vi "GenILCTestProf.vi"() -> ()   [LabVIEW 2016]
panel:
  in  "Offset [deg or mm]":dbl
  out "RUY Signals":T1
  in  "No Cycles":u16=3
  in  "Dwell Time [s]":dbl=1.0
  in  "Max Speed [/s]":dbl=5.0
  in  "Travel [deg or mm]":dbl=20.0
  in  "Select Joint No.":T2(ring)=enum."Joint 3"
  out "Joint 4 Graph":dbl[](graph)
  out "Joint 3 Graph":dbl[](graph)
  out "Joint 2 Graph":dbl[](graph)
  out "Joint 1 Graph":dbl[](graph)
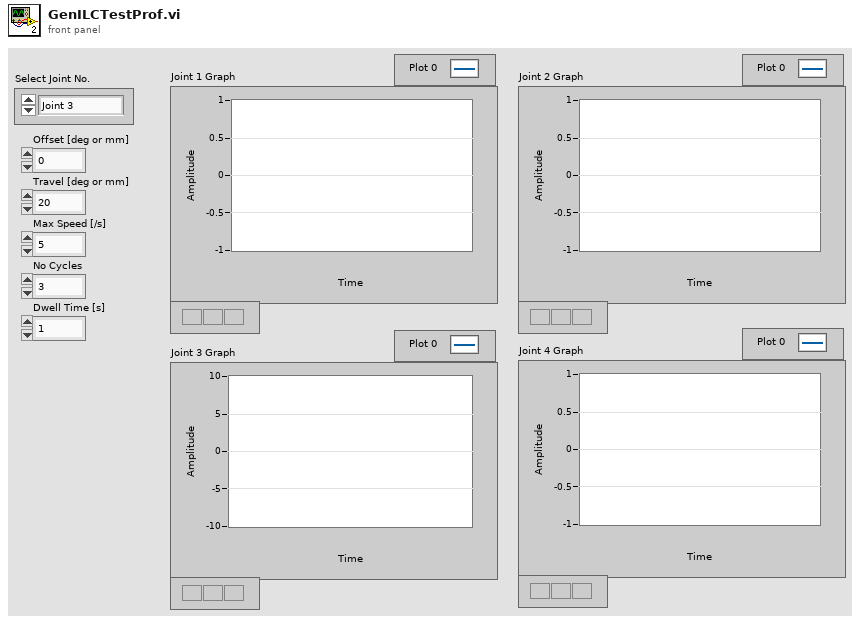
[diagram p1: front panel]
types:
  T1 = cluster{"Ref":cluster{"theta 1 Array":dbl[], "theta 2 Array":dbl[], "d3 Array":dbl[], "theta 4 Array":dbl[]}, "uFF":cluster{"theta 1 Array":dbl[], "theta 2 Array":dbl[], "d3 Array":dbl[], "theta 4 Array":dbl[]}, "yOut":cluster{"theta 1 Array":dbl[], "theta 2 Array":dbl[], "d3 Array":dbl[], "theta 4 Array":dbl[]}}
  T2 = enum16{"Joint 1", "Joint 2", "Joint 3", "Joint 4"}
  T3 = cluster{"theta 1 Array":dbl[], "theta 2 Array":dbl[], "d3 Array":dbl[], "theta 4 Array":dbl[]}
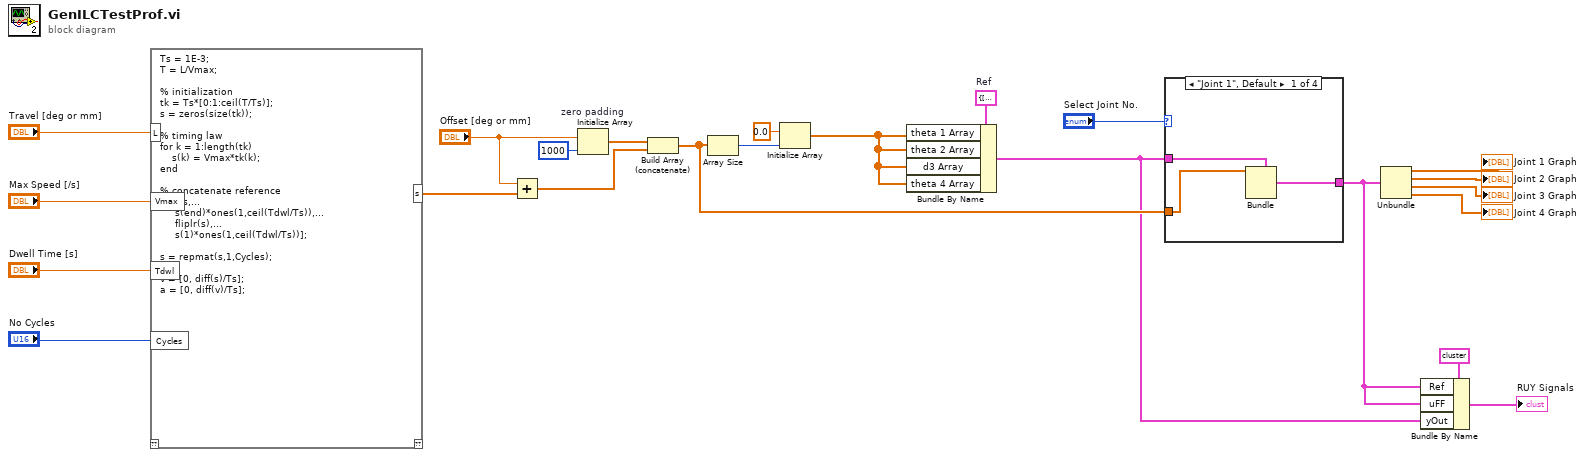
[diagram p0: block diagram]
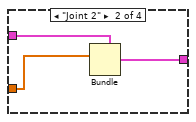
[diagram p2: hidden frame]
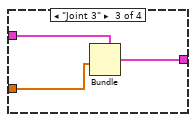
[diagram p3: hidden frame]
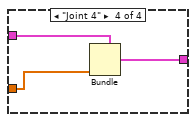
[diagram p4: hidden frame]
diagram:
  w15 = T3 {"theta 1 Array"=[], "theta 2 Array"=[], "d3 Array"=[], "theta 4 Array"=[]}  # Ref
  n1 = script code="Ts = 1E-3;\nT = L/Vmax;\n\n% initialization\ntk = Ts*[0:1:ceil(T/Ts)];\ns = zeros(size(tk));\n\n% timing law\nfor k = 1:length(tk) \n    s(k) = Vmax*tk(k);\nend\n\n% concatenate reference\ns = [s,...\n     s(end)*ones(1,ceil(Tdwl/Ts)),...\n     fliplr(s),...\n     s(1)*ones(1,ceil(Tdwl/Ts))];\n\ns = repmat(s,1,Cycles);\n\nv = [0, diff(s)/Ts];\na = [0, diff(v)/Ts];"("L"="Travel [deg or mm]", "Vmax"="Max Speed [/s]", "Tdwl"="Dwell Time [s]", "Cycles"="No Cycles") -> ("s"=w2:dbl[])  [unwired: 1 in, 1 out]
  n2 = Add(x="Offset [deg or mm]", y=w2) -> (x+y=w1:dbl[])
  n3 = Initialize Array "zero padding"("Offset [deg or mm]", 1000 ("dimension size")) -> (w4:dbl[])
  n4 = Build Array (concatenate)(w4, w1) -> (w9:dbl[])
  n5 = Array Size(array=w9) -> (size(s)=w19:i32)
  n6 = Initialize Array(0.0 ("element"), w19) -> (w17:dbl[])
  n7 = Bundle By Name(cluster=w15, "theta 1 Array"=w17, "theta 2 Array"=w17, "d3 Array"=w17, "theta 4 Array"=w17) -> (w8:T3)
  n8 = case shown="\"Joint 1\", Default" "Select Joint No." {
    tunnel: w8 -> [w26 w29 w32 w35]
    tunnel: w9 -> [w25 w28 w31 w34]
    tunnel: [w24 w27 w30 w33] -> w5
    frame "Joint 1", Default {
      n9 = Bundle(cluster=w26, "theta 1 Array"=w25) -> (w24:T3)  [unwired: 3 in]
    }
    frame "Joint 2" {
      n10 = Bundle(cluster=w29, "theta 2 Array"=w28) -> (w27:T3)  [unwired: 3 in]
    }
    frame "Joint 3" {
      n11 = Bundle(cluster=w32, "d3 Array"=w31) -> (w30:T3)  [unwired: 3 in]
    }
    frame "Joint 4" {
      n12 = Bundle(cluster=w35, "theta 4 Array"=w34) -> (w33:T3)  [unwired: 3 in]
    }
  }
  n13 = Unbundle(w5) -> ("theta 1 Array"=→"Joint 1 Graph":dbl[], "theta 2 Array"=→"Joint 2 Graph":dbl[], "d3 Array"=→"Joint 3 Graph":dbl[], "theta 4 Array"=→"Joint 4 Graph":dbl[])
  n14 = Bundle By Name(cluster=T1 {"Ref"={"theta 1 Array"=array[6000 elements], "theta 2 Array"=array[6000 elements], "d3 Array"=array[6000 elements], "theta 4 Array"=array[6000 elements]}, "uFF"={"theta 1 Array"=array[6000 elements], "theta 2 Array"=array[6000 elements], "d3 Array"=array[6000 elements], "theta 4 Array"=array[6000 elements]}, "yOut"={"theta 1 Array"=[0.0], "theta 2 Array"=[0.0], "d3 Array"=[0.0], "theta 4 Array"=[0.0]}} ("RUY Signals 2"), "Ref"=w5, "uFF"=w5, "yOut"=w8) -> (→"RUY Signals":T1)
